vi "Search.vi"(8 "error in (no error)":errorcluster caption="entrée d'erreur (pas d'erreur)", 11 "Firebase Benches en entrée":refnum<class "Firebase Find_Batch_Fct_SN.lvclass">) -> (0 "error out":errorcluster caption="sortie d'erreur", 3 "Firebase Benches en sortie":refnum<class "Firebase Find_Batch_Fct_SN.lvclass">)   [LabVIEW 2020, in "Library Instrument & Equipement.lvlib" / "Library FireBase.lvlib" / "Firebase Find_Batch_Fct_SN.lvclass"]
doc: "Returns data according to Value_To_Find on Collection_to_find Use Nb_To_Read to determine the number to read\nPlease initialise the following values before use the VI\n - Name BDD\n - Value to find\n - API Key\n - Field Filter\n - Field Order\n - Collection_to_find\n\nIf there is no Field order -> Field Order=Field Filter"
uses:
  Firebase Find_Batch_Fct_SN.lvclass
  C:/Users/ngarcin/OneDrive - Altyor/Standard TB/Class/Firebase/Source/Firebase Driver/Firebase Driver.lvclass
  Firebase Find_Batch_Fct_SN.lvclass/Firebase Find_Batch_Fct_SN.ctl
  JSON API/JSON Value/Set from JSON string.vi
  JSON API/JSON Value/JSON Value.lvclass
  JSON API/Variant JSON/Variant JSON.lvlib
  JSON API/Get Polymorphic/JSON GetSet.lvlib
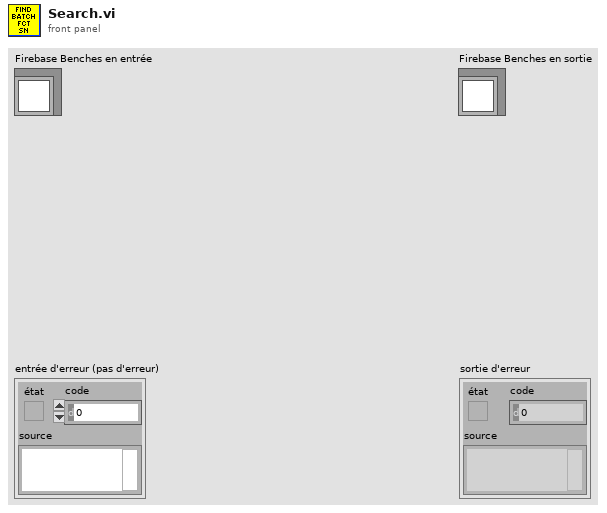
[diagram p1: front panel]
types:
  T1 = cluster{"name":string, "fields":cluster{"Result":cluster{"booleanValue":bool}, "CreationDate":cluster{"timestampValue":string}, "Batch":cluster{"stringValue":string}, "SerialNumber":cluster{"stringValue":string}, "EndOfProduction":cluster{"timestampValue":string}, "PartNumber":cluster{"stringValue":string}, "OrderNumber":cluster{"stringValue":string}, "Operator":cluster{"stringValue":string}}}[]
  T2 = cluster{"name":string, "fields":cluster{"Result":cluster{"booleanValue":bool}, "CreationDate":cluster{"timestampValue":string}, "Batch":cluster{"stringValue":string}, "SerialNumber":cluster{"stringValue":string}, "EndOfProduction":cluster{"timestampValue":string}, "PartNumber":cluster{"stringValue":string}, "OrderNumber":cluster{"stringValue":string}, "Operator":cluster{"stringValue":string}}}
  T3 = cluster{"document":cluster{"name":string, "fields":cluster{"Result":cluster{"booleanValue":bool}, "CreationDate":cluster{"timestampValue":string}, "Batch":cluster{"stringValue":string}, "SerialNumber":cluster{"stringValue":string}, "EndOfProduction":cluster{"timestampValue":string}, "PartNumber":cluster{"stringValue":string}, "OrderNumber":cluster{"stringValue":string}, "Operator":cluster{"stringValue":string}}}}
  T4 = cluster{"document":cluster{"name":string, "fields":cluster{"Result":cluster{"booleanValue":bool}, "CreationDate":cluster{"timestampValue":string}, "Batch":cluster{"stringValue":string}, "SerialNumber":cluster{"stringValue":string}, "EndOfProduction":cluster{"timestampValue":string}, "PartNumber":cluster{"stringValue":string}, "OrderNumber":cluster{"stringValue":string}, "Operator":cluster{"stringValue":string}}}}[]
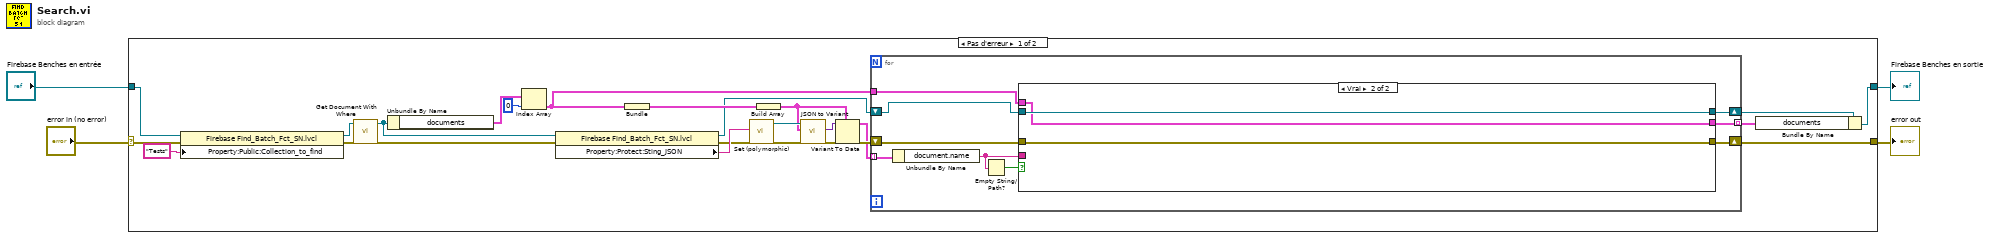
[diagram p0: block diagram]
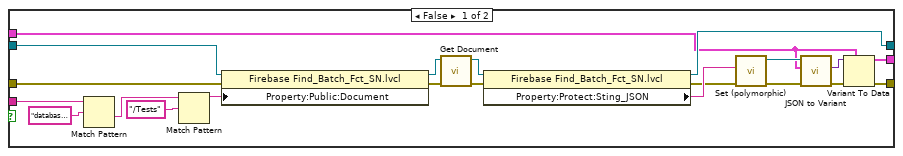
[diagram p2: hidden frame]
diagram:
  n1 = case shown="Pas d'erreur" "error in (no error)" {
    selector: "error in (no error)" -> [w19 w64]
    tunnel: "Firebase Benches en entrée" -> [w21 w63]
    tunnel: [w10 w64] -> w3
    tunnel: [w5 w63] -> w2
    frame No Error {
      n2 = property class="Firebase Find_Batch_Fct_SN.lvcl"(reference=w21, error in=w19, "Property:Public:Collection_to_find"="Tests" ("Collection_to_find")) -> (reference out=w15:refnum<class "Firebase Find_Batch_Fct_SN.lvclass">, error out=w18:errorcluster)
      n3 = call-dynamic "Get Document With Where.vi"("error in (no error)"=w18, "Firebase (Default) en entrée"=w15) -> ("error out"=w17:errorcluster, "Firebase (Default) en sortie"=w16:refnum<class "Firebase Find_Batch_Fct_SN.lvclass">)  [unwired: 8 in]
      n4 = Unbundle By Name(w16) -> ("documents"=w13:T1)
      n5 = Index Array(array=w13, index=0 ("indice")) -> (element=w9:T2)
      n6 = property class="Firebase Find_Batch_Fct_SN.lvcl"(reference=w16, error in=w17) -> (reference out=w8:refnum<class "Firebase Find_Batch_Fct_SN.lvclass">, error out=w23:errorcluster, "Property:Protect:Sting_JSON"=w26:string)
      n7 = Bundle("document"=w9) -> (w24:T3)  [unwired: 1 in]
      n8 = call-poly "Set (polymorphic).vi"("error in (no error)"=w23, "JSON stream"=w26) -> ("error out"=w27:errorcluster, "JSON Value out"=w29:refnum<class "JSON Value.lvclass">)  [unwired: 7 in, 1 out]
      n9 = Build Array(w24) -> (w14:T4)
      n10 = call "JSON to Variant.vi"("error in (no error)"=w27, "Variant (Data Type)"=w14, "JSON Value"=w29) -> ("error out"=w28:errorcluster, "Variant out"=w22:variant)  [unwired: 7 in]
      n11 = Variant To Data(error in=w28, type=w14, Variant=w22) -> (data=w11:T4, error out=w12:errorcluster)
      n12 = for {
        shift-right: [w35] -> w7
        shift-left: w8 -> [w38]
        shift-right: [w36] -> w10
        shift-left: w12 -> [w37]
        tunnel: w9 -> [w34]
        tunnel: [w33] -> w6 mode=indexing
        tunnel: w11 -> [w32] mode=indexing
        n13 = Unbundle By Name(w32) -> ("document.name"=w31:string)
        n14 = Empty String/Path?(string/path=w31) -> (empty?=w30:bool)
        n15 = case shown="Vrai" w30 {
          tunnel: w31 -> [w56 _]
          tunnel: w38 -> [w55 w62]
          tunnel: w37 -> [w52 w60]
          tunnel: [w44 w60] -> w36
          tunnel: [w42 w62] -> w35
          tunnel: w34 -> [w40 w61]
          tunnel: [w39 w61] -> w33
          frame False {
            n16 = Match Pattern(string=w56, regular expression="databases/(default)/documents/" ("expression régulière")) -> (after substring=w58:string)  [unwired: 1 in, 3 out]
            n17 = Match Pattern(string=w58, regular expression="/Tests" ("expression régulière")) -> (before substring=w41:string)  [unwired: 1 in, 3 out]
            n18 = property class="Firebase Find_Batch_Fct_SN.lvcl"(reference=w55, error in=w52, "Property:Public:Document"=w41) -> (reference out=w54:refnum<class "Firebase Find_Batch_Fct_SN.lvclass">, error out=w53:errorcluster)
            n19 = call-dynamic "Get Document.vi"("error in (no error)"=w53, "Firebase (Default) en entrée"=w54) -> ("error out"=w51:errorcluster, "Firebase (Default) en sortie"=w43:refnum<class "Firebase Find_Batch_Fct_SN.lvclass">)  [unwired: 8 in]
            n20 = property class="Firebase Find_Batch_Fct_SN.lvcl"(reference=w43, error in=w51) -> (reference out=w42:refnum<class "Firebase Find_Batch_Fct_SN.lvclass">, error out=w45:errorcluster, "Property:Protect:Sting_JSON"=w46:string)
            n21 = call-poly "Set (polymorphic).vi"("error in (no error)"=w45, "JSON stream"=w46) -> ("error out"=w49:errorcluster, "JSON Value out"=w47:refnum<class "JSON Value.lvclass">)  [unwired: 7 in, 1 out]
            n22 = call "JSON to Variant.vi"("error in (no error)"=w49, "Variant (Data Type)"=w40, "JSON Value"=w47) -> ("error out"=w48:errorcluster, "Variant out"=w50:variant)  [unwired: 7 in]
            n23 = Variant To Data(error in=w48, type=w40, Variant=w50) -> (data=w39:T2, error out=w44:errorcluster)
          }
          frame True {
          }
        }
      }
      n24 = Bundle By Name(cluster=w7, "documents"=w6) -> (w5:refnum<class "Firebase Find_Batch_Fct_SN.lvclass">)
    }
    frame Error {
    }
  }
  "error out" <- w3
  "Firebase Benches en sortie" <- w2
